vi "RemoteEventFGV.vi"(8 "Error In":errorcluster, 10 "Operation (Read)":enum16{"Read", "Write"}(ring), 11 "Remote Event in":T1) -> (0 "Error Out":errorcluster, 3 "Remote Event out":T1)   [LabVIEW 2020]
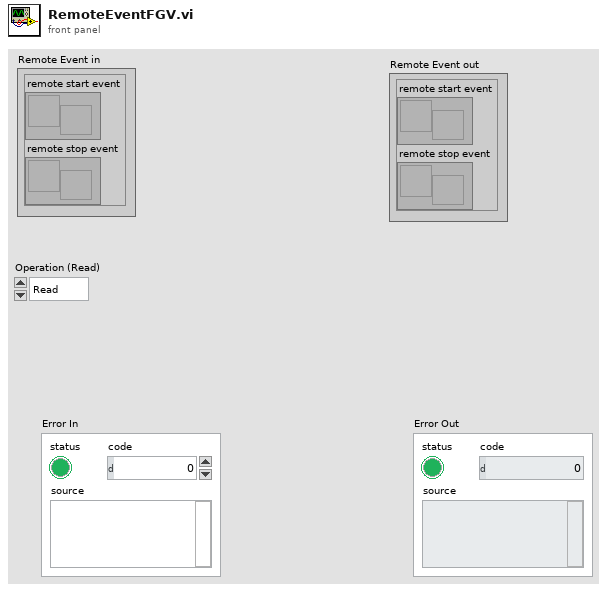
[diagram p1: front panel]
types:
  T1 = cluster{"remote start event":refnum<user-event>, "remote stop event":refnum<user-event>}
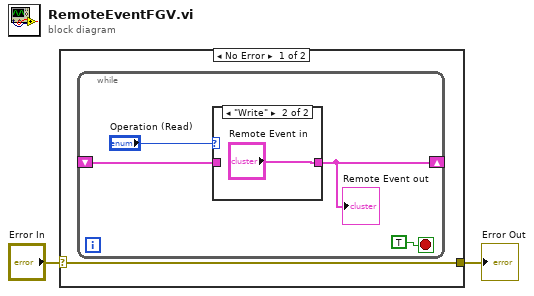
[diagram p0: block diagram]
diagram:
  n1 = case shown="No Error" "Error In" {
    selector: "Error In" -> [w3 w10]
    tunnel: [w3 w10] -> w1
    frame No Error {
      n2 = while {
        shift-right: [w4] -> _
        shift-left: _ -> [w5]
        stop <- TRUE stop-if-true
        n3 = case shown="\"Write\"" "Operation (Read)" {
          tunnel: [w8 "Remote Event in"] -> w4
          tunnel: w5 -> [w8 _]
          frame "Read", Default {
          }
          frame "Write" {
          }
        }
        "Remote Event out" <- w4
      }
    }
    frame Error {
    }
  }
  "Error Out" <- w1
